vi "Set Time Base.vi"(8 "error in (no error)":errorcluster, 11 "PicoScope 3000a in":refnum<class "PicoScope 3000a.lvclass">) -> (0 "error out":errorcluster, 3 "PicoScope 3000a out":refnum<class "PicoScope 3000a.lvclass">)   [LabVIEW 2018, in "PicoScope 3000a.lvlib" / "PicoScope 3000a.lvclass"]
uses:
  PicoScope 3000a.lvclass
  PicoScope 3000a.lvclass/PicoScope 3000a.ctl
  LWS SLA-070/Distro/Projects/12170 Luminar LWS Base/Source/PPLs/Configuration.lvlibp/Configuration.lvclass
  LWS SLA-070/Distro/Projects/12170 Luminar LWS Base/Source/PPLs/Oscilloscope.lvlibp/Oscilloscope.lvclass
  <instrlib>/PicoScope/PicoScope.lvlib
  C:/Projects/LWS SLA-070/Distro/Projects/12170 Luminar LWS Base/Source/PPLs/Oscilloscope.lvlibp/Oscilloscope.lvclass
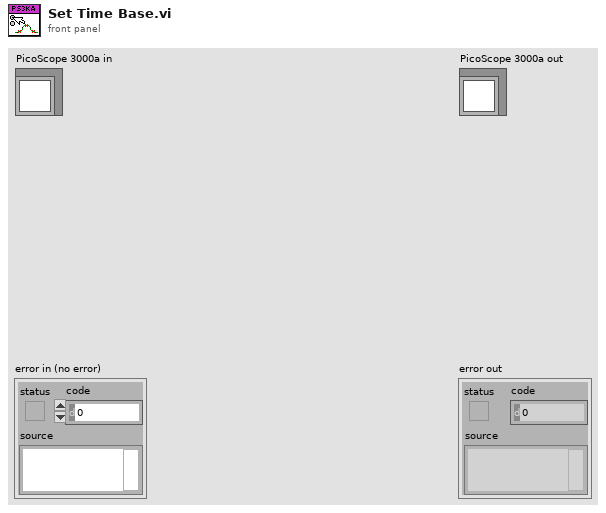
[diagram p1: front panel]
types:
  T1 = cluster{"preTriggerSamples":u32, "postTriggerSamples":u32, "timebase":u32, "Down-Sample Mode":i32, "Down Sample Ratio":u32}
  T2 = cluster{"Sample Frequency":sgl, "Sample Rate":sgl, "Max Samples Available":i32, "Number of Samples":u32, "Total Capture Time (sec) ":sgl, "Max Total Capture Time Available (sec)":sgl}
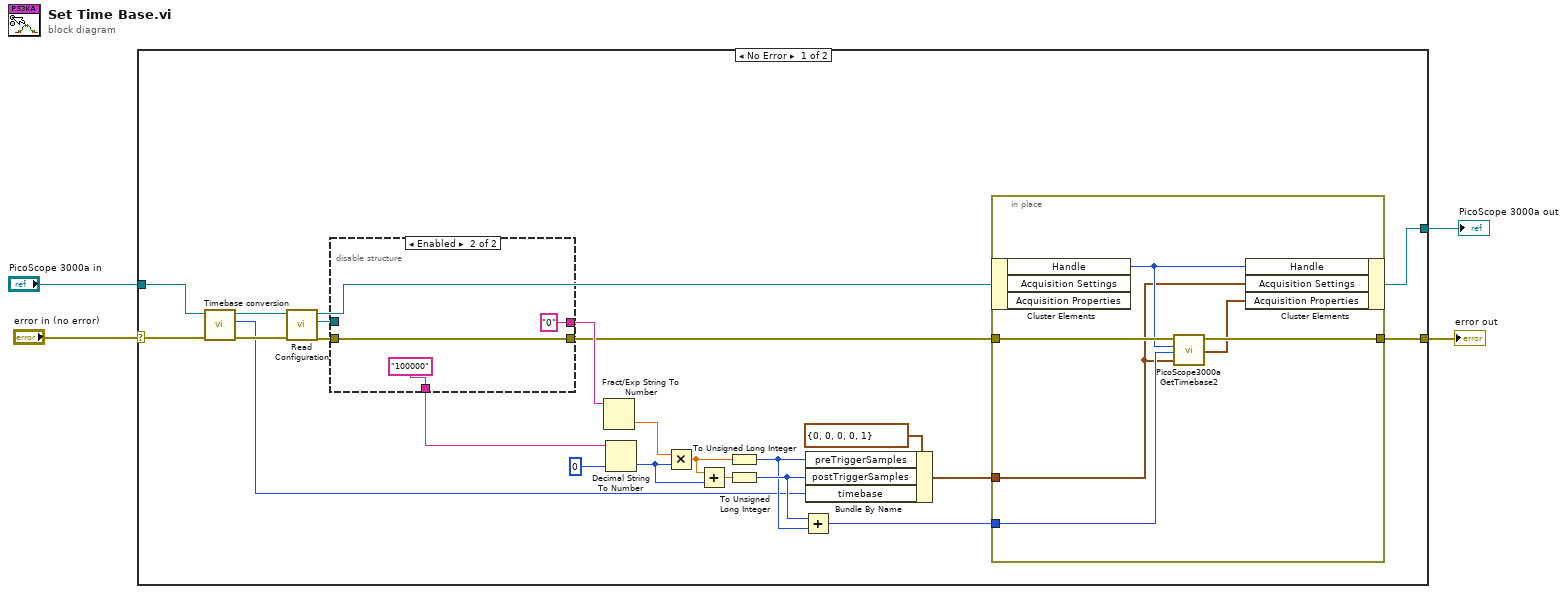
[diagram p0: block diagram]
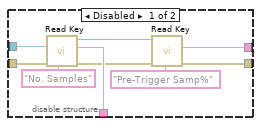
[diagram p2: hidden frame]
diagram:
  n1 = case shown="No Error" "error in (no error)" {
    selector: "error in (no error)" -> [w9 w47]
    tunnel: [w19 w47] -> w3
    tunnel: [w18 w46] -> w1
    tunnel: "PicoScope 3000a in" -> [w8 w46]
    frame No Error {
      n2 = call "Timebase conversion.vi"("error in (no error)"=w9, "PicoScope 3000a in"=w8) -> ("error out"=w6:errorcluster, "Timebase"=w5:u32, "PicoScope 3000a out"=w7:refnum<class "PicoScope 3000a.lvclass">)  [unwired: 7 in]
      n3 = call "Read Configuration.vi"("error in (no error)"=w6, "Oscilloscope in"=w7) -> ("error out"=w10:errorcluster, "Configuration"=w11:refnum<class "Configuration.lvclass">, "Oscilloscope out"=w22:refnum<class "PicoScope 3000a.lvclass">)  [unwired: 7 in]
      n4 = disable-structure shown="Enabled" {
        disable-tunnel: [w36 "100000" ("Value")] -> w27
        disable-tunnel: [w31 "0" ("Value")] -> w13
        disable-tunnel: [w30 w39] -> w12
        disable-tunnel: w11 -> [w29 _]
        disable-tunnel: w10 -> [w28 w39]
        frame Disabled {
          n5 = call "Read Key.vi"("Key:"="No. Samples", "error in"=w28, "Configuration in"=w29) -> ("error out"=w33:errorcluster, "Value"=w36:string, "Configuration out"=w32:refnum<class "Configuration.lvclass">)  [unwired: 6 in]
          n6 = call "Read Key.vi"("Key:"="Pre-Trigger Samp%", "error in"=w33, "Configuration in"=w32) -> ("error out"=w30:errorcluster, "Value"=w31:string)  [unwired: 6 in, 1 out]
        }
        frame Enabled {
        }
      }
      n7 = Fract/Exp String To Number(string=w13) -> (number=w14:dbl)  [unwired: 3 in, 1 out]
      n8 = Decimal String To Number(string=w27, default (0L)=u32 0 ("default (0 I32)")) -> (number=w21:u32)  [unwired: 1 in, 1 out]
      n9 = Multiply(x=w14, y=w21) -> (x*y=w25:dbl)
      n10 = Add(x=w25, y=w21) -> (x+y=w24:dbl)
      n11 = To Unsigned Long Integer(number=w25) -> (unsigned 32bit integer=w16:u32)
      n12 = To Unsigned Long Integer(number=w24) -> (unsigned 32bit integer=w17:u32)
      n13 = Add(x=w17, y=w16) -> (x+y=w15:u32)
      n14 = Bundle By Name(cluster=T1 {"preTriggerSamples"=0, "postTriggerSamples"=0, "timebase"=0, "Down-Sample Mode"=0, "Down Sample Ratio"=1} ("Acquisition Settings"), "preTriggerSamples"=w16, "postTriggerSamples"=w17, "timebase"=w5) -> (w23:T1)
      n15 = in-place {
        in-place-border: w12 -> [w45]
        in-place-border: w23 -> [w41]
        in-place-border: w15 -> [w43]
        in-place-border: [w42] -> w19
        n16 = in-place-cluster #1(w22) -> ("Handle"=w44:i16)  [unwired: 2 out]
        n17 = call <instrlib>:"PicoScope3000aGetTimebase2.vi"("Number of Samples"=w43, "Acquisition Settings"=w41, "handle in"=w44, "error in (no error)"=w45) -> ("error out"=w42:errorcluster, "Properties Panel"=w40:T2)  [unwired: 5 in, 1 out]
        n18 = in-place-cluster #1("Handle"=w44, "Acquisition Settings"=w41, "Acquisition Properties"=w40) -> (w18:refnum<class "PicoScope 3000a.lvclass">)
      }
    }
    frame Error {
    }
  }
  "error out" <- w3
  "PicoScope 3000a out" <- w1
